vi "solar_tcp Core.vi"(6 "Suppress Errors? (T)":bool=TRUE, 7 "Action":T4, 8 "error in (no error)":errorcluster, 9 "Read Timeout (0ms)":i32, 10 "Message to Send":string, 11 "TCP Data in":T1={"Connected"=FALSE, "Config"={"TCPServer"=enum."SERVER", "ServerPort"=0, "IPAddress"="", "ClientPort"=0, "HdrSizeBytes"=4, "HdrLenSubtractBytes"=0, "HdrLenOffsetBits"=0, "HdrLenSizeBits"=32}, "Clients"=[], "ConnectionID"=refnum, "Debug"=[]} {"Debug"."Time" format="%<%Y-%m-%d\n%H:%M:%S%3u>T"}) -> (0 "error out":errorcluster, 1 "Connected":bool, 2 "Message Read/Sent":string, 3 "TCP Data out":T1 {"Debug"."Time" format="%<%Y-%m-%d\n%H:%M:%S%3u>T"})   [LabVIEW 2018]
doc: "This is the TCP Server or Client core state machine that handles a TCP session. The <b>Message to Send</b> and <b>Message Read</b> should contain the entire TCP message including the header. Before writing the <b>Message to Send</b> the length field is updated as defined by the configuration header length offset and size. The total length field is typically the first 4 bytes of the message which includes the total packet size."
uses:
  solar_tcp_ctl Action.ctl
  solar_tcp_ctl Data.ctl
  solar_tcp_ctl Config.ctl
  solar_tcp_ctl Debug.ctl
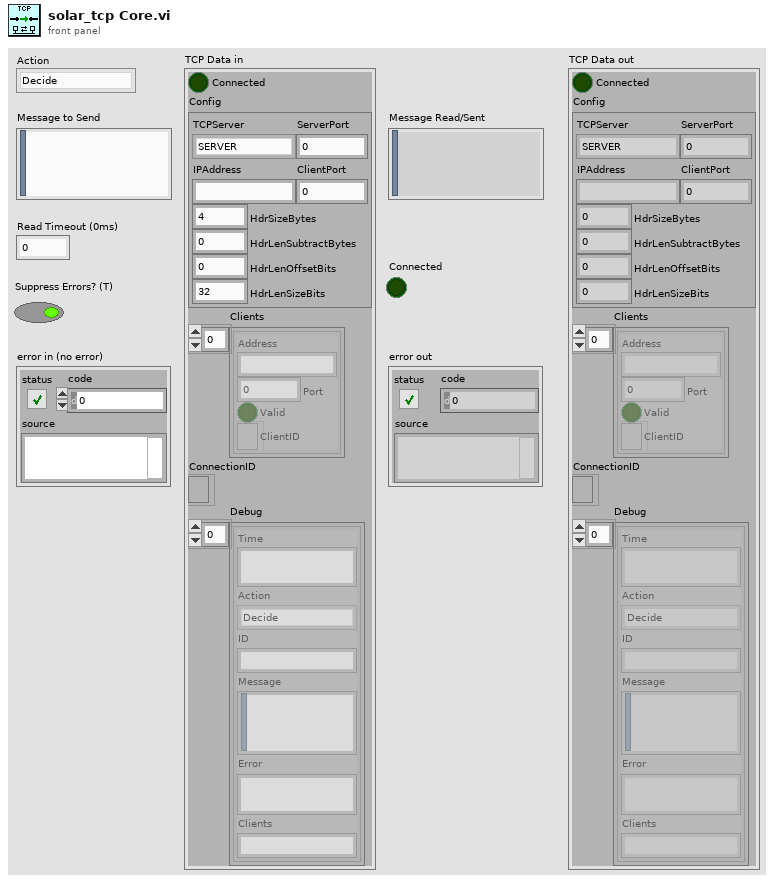
[diagram p1: front panel]
types:
  T1 = typedef "solar_tcp_ctl Data.ctl" = cluster{"Connected":bool, "Config":T2, "Clients":cluster{"Address":string, "Port":u16, "Valid":bool, "ClientID":refnum<k5>}[], "ConnectionID":refnum<k5>, "Debug":T3[]}
  T2 = typedef "solar_tcp_ctl Config.ctl" = cluster{"TCPServer":enum8{"SERVER", "CLIENT"}, "ServerPort":u16, "IPAddress":string, "ClientPort":u16, "HdrSizeBytes":i32, "HdrLenSubtractBytes":i32, "HdrLenOffsetBits":i32, "HdrLenSizeBits":i32}
  T3 = typedef "solar_tcp_ctl Debug.ctl" = cluster{"Time":timestamp, "Action":T4, "ID":string, "Message":string, "Error":string, "Clients":string}
  T4 = typedef "solar_tcp_ctl Action.ctl" = enum16{"Decide", "CreateListener", "Open", "Read", "Write", "Close", "Shutdown", "Done", "ChangePort"}
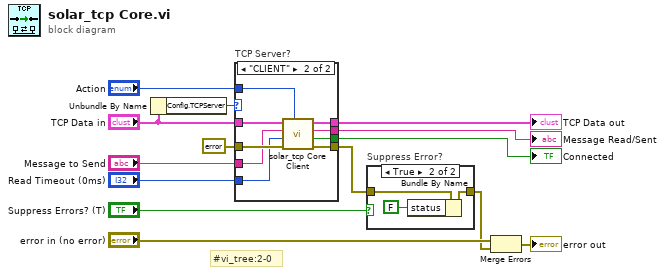
[diagram p0: block diagram]
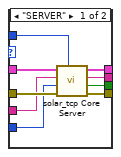
[diagram p2: hidden frame]
diagram:
  # "#vi_tree:2-0"
  n1 = Unbundle By Name("TCP Data in") -> ("Config.TCPServer"=w8:enum8{"SERVER", "CLIENT"})
  n2 = case "TCP Server?" shown="\"CLIENT\"" w8 {
    tunnel: [w16 w25] -> w14
    tunnel: "Action" -> [w21 w28]
    tunnel: "Message to Send" -> [w20 w30]
    tunnel: "TCP Data in" -> [w22 w31]
    tunnel: errorcluster {"status"=FALSE, "code"=0, "source"=""} ("error IO") -> [w23 w32]
    tunnel: [w18 w26] -> w10
    tunnel: [w17 w27] -> w5
    tunnel: [w15 w24] -> w9
    tunnel: "Read Timeout (0ms)" -> [w19 w29]
    frame "SERVER" {
      n3 = call "solar_tcp Core Server.vi"("Action"=w21, "error in (no error)"=w23, "Read Timeout (0ms)"=w19, "Message to Send"=w20, "TCP Data in"=w22) -> ("error out"=w17:errorcluster, "Connected"=w15:bool, "Message Read/Sent"=w16:string, "TCP Data out"=w18:T1)  [unwired: 3 in]
    }
    frame "CLIENT" {
      n4 = call "solar_tcp Core Client.vi"("Action"=w28, "error in (no error)"=w32, "Read Timeout (0ms)"=w29, "Message to Send"=w30, "TCP Data in"=w31) -> ("error out"=w27:errorcluster, "Connected"=w24:bool, "Message Read/Sent"=w25:string, "TCP Data out"=w26:T1)  [unwired: 3 in]
    }
  }
  "Message Read/Sent" <- w14
  "TCP Data out" <- w10
  "Connected" <- w9
  n5 = case "Suppress Error?" shown="True" "Suppress Errors? (T)" {
    tunnel: w5 -> [w33 w36]
    tunnel: [w33 w35] -> w2
    frame False {
    }
    frame True {
      n6 = Bundle By Name(cluster=w36, "status"=FALSE) -> (w35:errorcluster)
    }
  }
  n7 = Merge Errors("error in (no error)", w2) -> (→"error out":errorcluster)
